vi "Main.vi"() -> ()   [LabVIEW 2015]
doc: "The myRIO Project template acquires acceleration data from the onboard accelerometer and displays the changes of acceleration values in a waveform chart."
uses:
  <vilib>/myRIO/Instrument Drivers/Utilities/Utilities.lvlib
panel:
  in  "Error In":errorcluster
  in  "Rings":i32=3
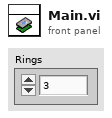
[diagram p1: front panel]
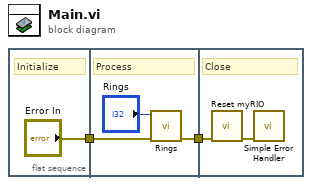
[diagram p0: block diagram]
diagram:
  n1 = flat-sequence {
    tunnel: ["Error In"] -> w1
    tunnel: [w6] -> w2
    tunnel: w1 -> [w5]
    tunnel: w2 -> [w7]
    frame #0 {
      # "Initialize"
    }
    frame #1 {
      # "Process"
      n2 = call "Rings.vi"("error in (no error)"=w5, "Rings"="Rings") -> ("error out"=w6:errorcluster)  [unwired: 9 in]
    }
    frame #2 {
      # "Close"
      n3 = call <vilib>:"Reset myRIO.vi"("error in (no error)"=w7) -> ("error out"=w8:errorcluster)  [unwired: 10 in]
      n4 = call <vilib>:"Simple Error Handler.vi"("error in (no error)"=w8) -> ()  [unwired: 4 in, 5 out]
    }
  }
